vi "Do.vi"(8 "error in (no error)":errorcluster, 9 "Events":refnum<class "Events.lvclass">, 10 "Message Loop Data in":T1, 11 "IInternalRequest in":refnum<class "IHandledUnsubscribed.lvclass">) -> (0 "error out":errorcluster, 2 "Message Loop Data out":T1, 3 "IInternalRequest out":refnum<class "IHandledUnsubscribed.lvclass">)   [LabVIEW 2020, in "wamplv.lvlib" / "IHandledUnsubscribed.lvclass"]
uses:
  IHandledUnsubscribed.lvclass
  Message loop classes/ErrorOrSuccess/ErrorOrSuccess.lvclass
  C:/local/wamplv/Private/Requests/IGenericInternalMessage/IGenericInternalMessage.lvclass
  C:/local/wamplv/Private/Requests/IInternalMessage/IInternalMessage.lvclass
  C:/local/wamplv/Private/Requests/MessageReceivedHandlers/Unsubscribed/IHandledUnsubscribed/IHandledUnsubscribed.lvclass
  wamplv.lvlib
  Unsubscribe/IUnsubscribe/IUnsubscribe.lvclass
  Message loop classes/Subscription details/SubscriptionDetailsParent/SubscriptionDetailsParent.lvclass
  WAMP Client/Private/TypeDef/Publish Requests Map.ctl
  WAMP Client/Private/TypeDef/Endpoint Data.ctl
  Call/ICallRequest/ICallRequest.lvclass
  WAMP Client/Private/TypeDef/CALL Request Map.ctl
  WAMP Client/Private/TypeDef/SUBSCRIBE Requests Map.ctl
  WAMP Client/Private/TypeDef/Subscriptions Map.ctl
  WAMP Client/Private/TypeDef/Unsubscribe Requests Map.ctl
  WAMP Client/Private/TypeDef/Unregister requests map.ctl
  WAMP Client/Private/TypeDef/Message Loop Data.ctl
  Events/EventsParent/Events.lvclass
  Subscribe/ISubscribe/ISubscribe.lvclass
  Publish/IPublish/IPublish.lvclass
  Register/IRegister/IRegister.lvclass
  Unregister/IUnregister/IUnregister.lvclass
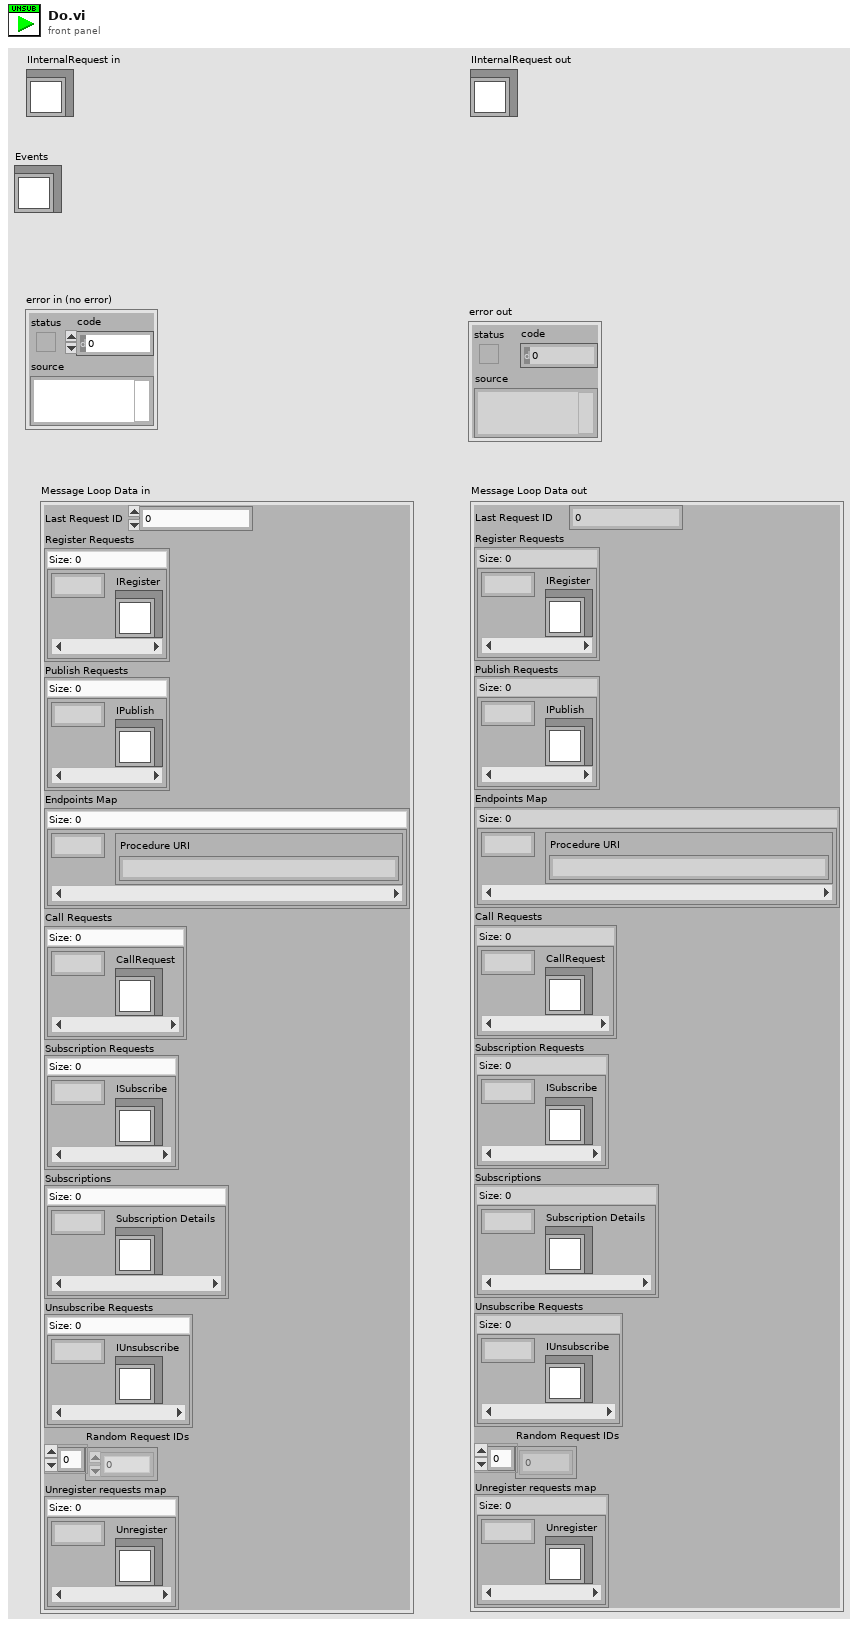
[diagram p1: front panel]
types:
  T1 = typedef "wamplv.lvlib/Message Loop Data.ctl" = cluster{"Last Request ID":u64, "Register Requests":map{u64, refnum<class "IRegister.lvclass">}, "Publish Requests":T2, "Endpoints Map":map{u64, T3}, "Call Requests":T4, "Subscription Requests":T5, "Subscriptions":T6, "Unsubscribe Requests":T7, "Random Request IDs":u64[], "Unregister requests map":T8}
  T2 = typedef "wamplv.lvlib/Publish Requests Map.ctl" = map{u64, refnum<class "IPublish.lvclass">}
  T3 = typedef "wamplv.lvlib/Endpoint Data.ctl" = cluster{"Procedure URI":string}
  T4 = typedef "wamplv.lvlib/CALL Request Map.ctl" = map{u64, refnum<class "ICallRequest.lvclass">}
  T5 = typedef "wamplv.lvlib/SUBSCRIBE Requests Map.ctl" = map{u64, refnum<class "ISubscribe.lvclass">}
  T6 = typedef "wamplv.lvlib/Subscriptions Map.ctl" = map{u64, refnum<class "SubscriptionDetailsParent.lvclass">}
  T7 = typedef "wamplv.lvlib/Unsubscribe Requests Map.ctl" = map{u64, refnum<class "IUnsubscribe.lvclass">}
  T8 = typedef "wamplv.lvlib/Unregister requests map.ctl" = map{u64, refnum<class "IUnregister.lvclass">}
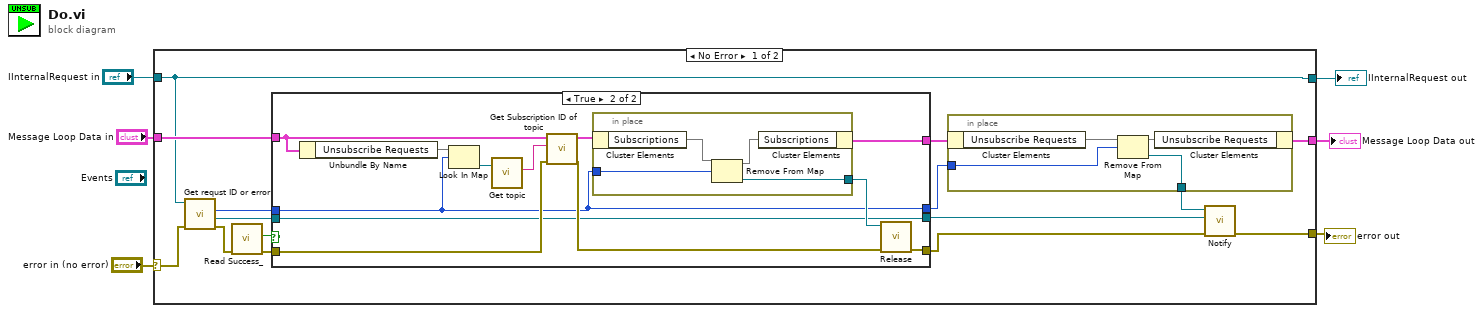
[diagram p0: block diagram]
diagram:
  n1 = case shown="No Error" "error in (no error)" {
    selector: "error in (no error)" -> [w21 w46]
    tunnel: "Message Loop Data in" -> [w18 w47]
    tunnel: [w9 w46] -> w4
    tunnel: [w8 w47] -> w3
    tunnel: "IInternalRequest in" -> [w7 w48]
    tunnel: [w7 w48] -> w1
    frame No Error {
      n2 = call-dynamic "Get requst ID or error.vi"("error in (no error)"=w21, "IHandledUnsubscribed in"=w7) -> ("error out"=w20:errorcluster, "ErrorOrSuccess"=w15:refnum<class "ErrorOrSuccess.lvclass">, "Unsubscription Request ID"=w17:u64)  [unwired: 6 in, 1 out]
      n3 = call "Read Success_.vi"("error in (no error)"=w20) -> ("error out"=w16:errorcluster, "Success?"=w19:bool)  [unwired: 8 in, 1 out]
      n4 = case shown="True" w19 {
        tunnel: w18 -> [w25 w36]
        tunnel: w17 -> [w22 w28]
        tunnel: w16 -> [w24 w31]
        tunnel: [w25 w29] -> w14
        tunnel: [w24 w27] -> w11
        tunnel: [w22 w28] -> w13
        tunnel: [w23 w26] -> w10
        tunnel: w15 -> [w23 w26]
        frame False {
        }
        frame True {
          n5 = Unbundle By Name(w36) -> ("Unsubscribe Requests"=w37:T7)
          n6 = Look In Map(map=w37, key=w28) -> (value=w35:refnum<class "IUnsubscribe.lvclass">)  [unwired: 1 in, 1 out]
          n7 = call-dynamic "Get topic.vi"("IUnsubscribe in"=w35) -> ("Topic URl"=w34:string)  [unwired: 9 in, 1 out]
          n8 = call "Get Subscription ID of topic.vi"("error in"=w31, "Topic"=w34, "Message loop data (in)"=w36) -> ("error out"=w30:errorcluster, "Message loop data (out)"=w33:T1)  [unwired: 6 in, 1 out]
          n9 = in-place {
            in-place-border: w28 -> [w41]
            in-place-border: [w38] -> w32
            n10 = in-place-cluster #1(w33) -> ("Subscriptions"=w40:T6)
            n11 = Remove From Map(10:w41, 11:w40) -> (1:w38:refnum<class "SubscriptionDetailsParent.lvclass">, 3:w39:T6)  [unwired: 1 out]
            n12 = in-place-cluster #1("Subscriptions"=w39) -> (w29:T1)
          }
          n13 = call-dynamic "Release.vi"("error in (no error)"=w30, "SubscriptionDetailsParent in"=w32) -> ("error out"=w27:errorcluster)  [unwired: 8 in, 1 out]
        }
      }
      n14 = in-place "In Place Element Structure" {
        in-place-border: w13 -> [w45]
        in-place-border: [w44] -> w12
        n15 = in-place-cluster #2(w14) -> ("Unsubscribe Requests"=w43:T7)
        n16 = Remove From Map(10:w45, 11:w43) -> (1:w44:refnum<class "IUnsubscribe.lvclass">, 3:w42:T7)  [unwired: 1 out]
        n17 = in-place-cluster #2("Unsubscribe Requests"=w42) -> (w8:T1)
      }
      n18 = call-dynamic "Notify.vi"("error in (no error)"=w11, "ErrorOrSuccess"=w10, "IUnsubscribe in"=w12) -> ("error out"=w9:errorcluster)  [unwired: 7 in, 1 out]
    }
    frame Error {
    }
  }
  "error out" <- w4
  "IInternalRequest out" <- w1
  "Message Loop Data out" <- w3
